vi "HapticSPM_read.vi"() -> ()   [LabVIEW 2017]
uses:
  Program Files/National Instruments/LabVIEW 2019/user.lib/HapticSTM/HapticSTM.lvlib
  Program Files/National Instruments/LabVIEW 2019/user.lib/Nanonis Prog Interface V5/Nanonis Prog Interface.lvlib
panel:
  in  "Reset Button":bool
  in  "Fine Adjust":dbl(slide)=3.163265306122449 scale=0.0..10.0
  out "Value":sgl format="%.1p"
  in  "Index":i8
  out "Size (m)":cluster{"Width":sgl, "Height":sgl} {"Height" format="%.1p"; "Width" format="%.1p"}
  out "Origin (m)":cluster{"Xc":sgl, "Yc":sgl} {"Yc" format="%.1p"; "Xc" format="%.1p"}
  out "Positions":T1 {"z (mm)" format="%.1p"; "y (nm)" format="%.1p"; "x (nm)" format="%.1p"}
  out "Forces":T2 {"Fz (N)" format="%.1f"; "Fy (N)" format="%.1f"; "Fx (N)" format="%.1f"}
  in  "Save":bool
  out "Arm Output:":dbl format="%^.1g"
  in  "Rough Adjust":dbl
  in  "Drag":dbl=1.0
  in  "STOP":bool
  out "Clicks":dbl
  # "Read Mode - Haptic SPM"
  # "Signal"
  # "Sensitivity"
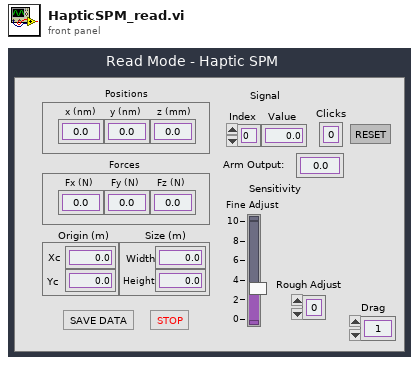
[diagram p1: front panel]
types:
  T1 = cluster{"x (nm)":dbl, "y (nm)":dbl, "z (mm)":dbl}
  T2 = cluster{"Fx (N)":dbl, "Fy (N)":dbl, "Fz (N)":dbl}
  T3 = cluster{"Xc":dbl, "Yc":dbl, "Width":dbl, "Height":dbl}
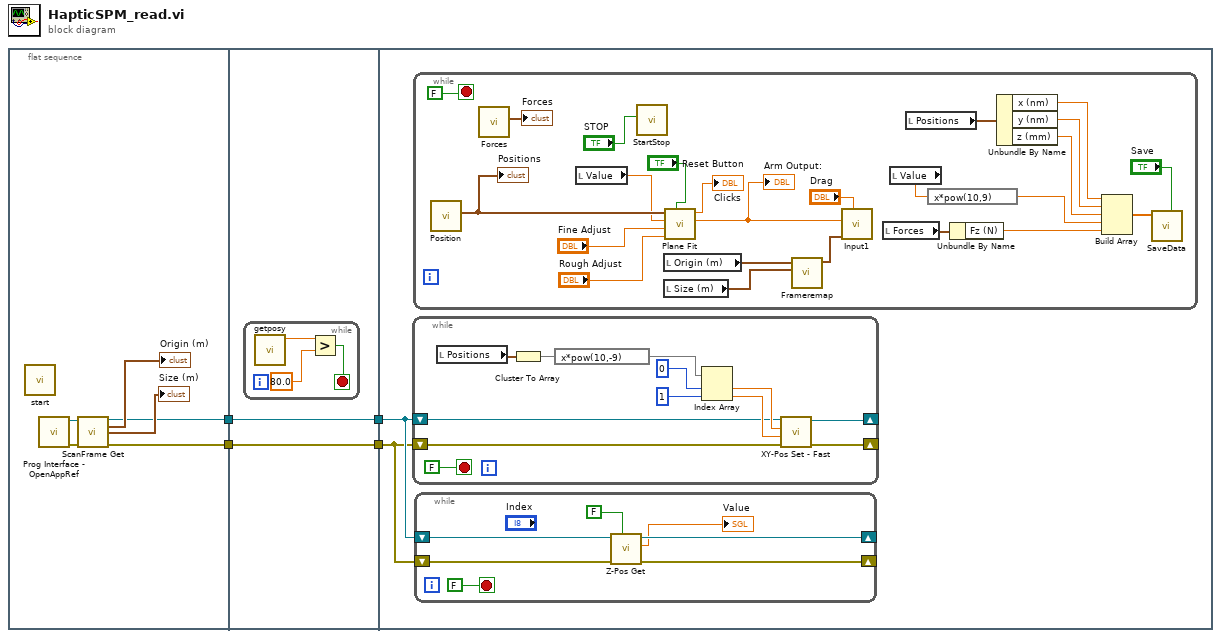
[diagram p0: block diagram]
diagram:
  n1 = flat-sequence {
    tunnel: [w6] -> w3
    tunnel: [w5] -> w1
    tunnel: [w12] -> w4
    tunnel: w3 -> [w12]
    tunnel: [w11] -> w2
    tunnel: w1 -> [w11]
    tunnel: w4 -> [w17]
    tunnel: w2 -> [w16]
    frame #0 {
      n2 = call "start.vi"() -> ()  [unwired: 11 in, 1 out]
      n3 = call <userlib>:"Prog Interface - OpenAppRef.vi"() -> ("Error out"=w9:errorcluster, "Application reference"=w10:refnum<vi>)  [unwired: 6 in]
      n4 = call <userlib>:"ScanFrame Get.vi"("Application ref in"=w10, "error in (no error)"=w9) -> ("Application ref out"=w6:refnum<vi>, "Center coordinates (m)"=→"Origin (m)":cluster{"Xc":sgl, "Yc":sgl}, "Size (m)"=→"Size (m)":cluster{"Width":sgl, "Height":sgl}, "error out"=w5:errorcluster)  [unwired: 9 in, 1 out]
    }
    frame #1 {
      n5 = while {
        stop <- w13 stop-if-true
        n6 = call "getposy.vi"() -> ("function return"=w15:dbl)  [unwired: 11 in]
        n7 = Greater?(x=w15, y=80.0) -> (0:w13:bool)
      }
    }
    frame #2 {
      n8 = while {
        shift-right: [w26] -> _
        shift-left: w17 -> [w28]
        shift-right: [w25] -> _
        shift-left: w16 -> [w27]
        stop <- FALSE stop-if-true
        n9 = local read "Positions"() -> (w35:T1)
        n10 = Cluster To Array(cluster=w35) -> (array=w34:dbl[])
        n11 = expression code="x*pow(10,-9)"(w34) -> (w33:dbl[])
        n12 = Index Array(array=w33, index #1=0 ("index"), index #2=1 ("index")) -> (element #1=w30:dbl, element #2=w29:dbl)
        n13 = call <userlib>:"XY-Pos Set - Fast.vi"("error in (no error)"=w27, "Y (m)"=w29, "X (m)"=w30, "Application ref in"=w28) -> ("error out"=w25:errorcluster, "Application ref out"=w26:refnum<vi>)  [unwired: 5 in]
      }
      n14 = while {
        stop <- FALSE stop-if-true
        n15 = call "Position.vi"() -> ("Positions"=w56:T1)  [unwired: 11 in]
        "Positions" <- w56
        n16 = call "Forces.vi"() -> ("Forces"=→"Forces":T2)  [unwired: 11 in]
        n17 = local read "Value"() -> (w54:sgl)
        n18 = call "StartStop.vi"("STOP"="STOP") -> ()  [unwired: 11 in]
        n19 = local read "Origin (m)"() -> (w53:cluster{"Xc":sgl, "Yc":sgl})
        n20 = local read "Size (m)"() -> (w52:cluster{"Width":sgl, "Height":sgl})
        n21 = call "Plane Fit.vi"("Reset Button"="Reset Button", "Rough Adjust"="Rough Adjust", "Fine Adjust"="Fine Adjust", "Nano Z"=w54, "Positions"=w56) -> ("Output"=w41:dbl, "Clicks"=→"Clicks":dbl)  [unwired: 5 in]
        "Arm Output:" <- w41
        n22 = call "Frameremap.vi"("Size (m)"=w52, "Origin (m)"=w53) -> ("Remapped Frame Properties"=w40:T3)  [unwired: 9 in]
        n23 = call "Input1.vi"("Drag"="Drag", "Remapped Frame Properties"=w40, "Signal in"=w41) -> ()  [unwired: 9 in]
        n24 = local read "Forces"() -> (w44:T2)
        n25 = local read "Value"() -> (w46:sgl)
        n26 = local read "Positions"() -> (w50:T1)
        n27 = expression code="x*pow(10,9)"(w46) -> (w45:sgl)
        n28 = Unbundle By Name(w44) -> ("Fz (N)"=w43:dbl)
        n29 = Unbundle By Name(w50) -> ("x (nm)"=w49:dbl, "y (nm)"=w48:dbl, "z (mm)"=w47:dbl)
        n30 = Build Array(w49, w48, w47, w45, w43) -> (w42:dbl[])
        n31 = call "SaveData.vi"("Save"="Save", "Data"=w42) -> ()  [unwired: 10 in]
      }
      n32 = while {
        shift-right: [w21] -> _
        shift-left: w17 -> [w24]
        shift-right: [w20] -> _
        shift-left: w16 -> [w23]
        stop <- FALSE stop-if-true
        n33 = call <userlib>:"Z-Pos Get.vi"("Wait for newest data (F=False)"=FALSE, "error in (no error)"=w23, "Application ref in"=w24) -> ("error out"=w20:errorcluster, "Z position (m)"=→"Value":sgl, "Application ref out"=w21:refnum<vi>)  [unwired: 6 in]
      }
    }
  }
